vi "step.vi"(0 "Desired Position":i32, 1 "Current Position":i32, 4 "stop":bool) -> (2 "Position Out":i32, 3 "Sensor Head Position":i32)   [LabVIEW 2014]
panel:
  out "error out":errorcluster
  out "Done":bool
  out "Gauge":i32(knob)
  out "Loop Number":i32
  # "In stepper \nmotor steos"
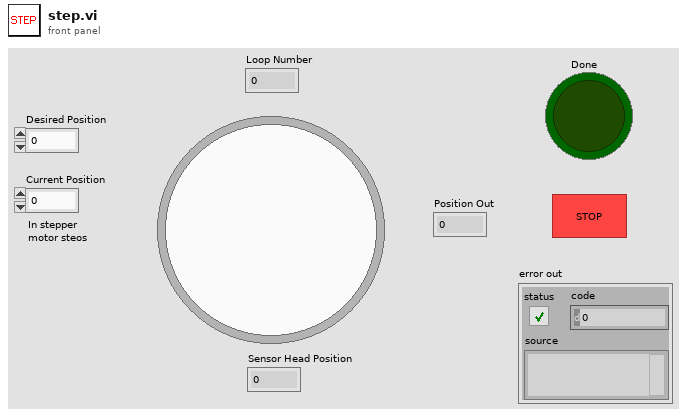
[diagram p1: front panel]
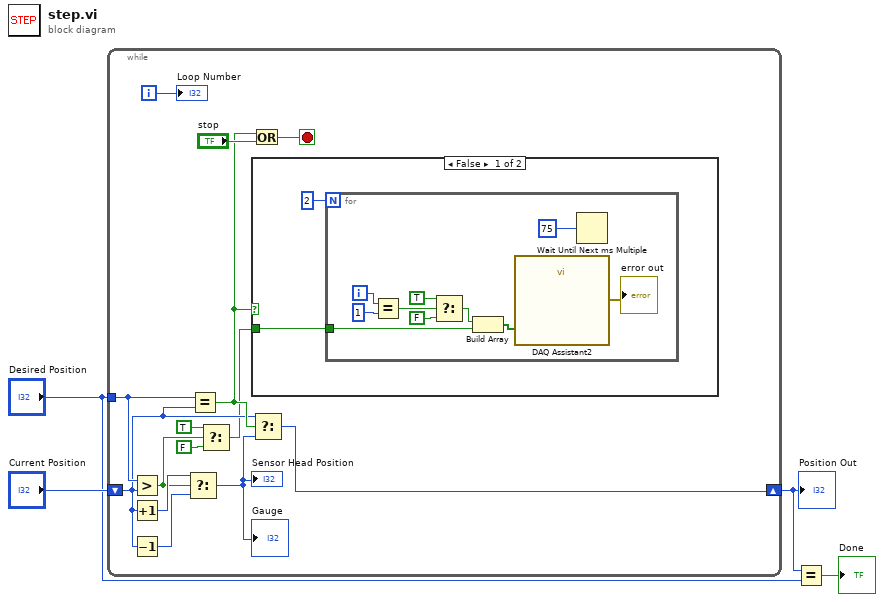
[diagram p0: block diagram]
diagram:
  n1 = while {
    shift-right: [w15] -> w3
    shift-left: "Current Position" -> [w12]
    tunnel: "Desired Position" -> [w13]
    i -> [w18]
    stop <- w17 stop-if-true
    n2 = Greater?(x=w13, y=w12) -> (0:w6:bool)
    n3 = Increment(x=w12) -> (x+1=w10:i32)
    n4 = Decrement(x=w12) -> (x-1=w11:i32)
    n5 = Select(t=w10, s=w6, f=w11) -> (s? t:f=w5:i32)
    "Gauge" <- w5
    "Sensor Head Position" <- w5
    n6 = Equal?(x=w13, y=w12) -> (x = y?=w14:bool)
    n7 = Select(t=TRUE, s=w6, f=FALSE) -> (s? t:f=w7:bool)
    n8 = Or(x=w14, y="stop") -> (x .or. y?=w17:bool)
    n9 = case shown="False" w14 {
      tunnel: w7 -> [w19 _]
      frame False {
        n10 = for {
          N: 2 -> [_]
          tunnel: w19 -> [w24]
          i -> [w29]
          n11 = Equal?(x=w29, y=1) -> (x = y?=w28:bool)
          n12 = Select(t=TRUE, s=w28, f=FALSE) -> (s? t:f=w25:bool)
          n13 = Build Array(w25, w24) -> (w23:bool[])
          n14 = call "DAQ Assistant2"("data"=w23) -> ("error out"=→"error out":errorcluster)  [unwired: 17 in, 1 out]
          n15 = Wait Until Next ms Multiple(millisecond multiple=75) -> ()  [unwired: 1 out]
        }
      }
      frame True {
        # "If Desired = Current, don't step the motor"
      }
    }
    n16 = Select(t=w12, s=w14, f=w5) -> (s? t:f=w15:i32)
    "Loop Number" <- w18
  }
  "Position Out" <- w3
  n17 = Equal?(x=w3, y="Desired Position") -> (x = y?=→"Done":bool)
